vi "Find max pump WP angle.vi"(8 "error in (no error)":errorcluster, 9 "Angle":dbl, 10 "Delay":u32, 11 "VISA Refnum in":refnum<visa-resource-name>) -> (0 "error out":errorcluster, 1 "Numeric":dbl, 2 "Current position (units)":dbl, 3 "VISA Refnum out":refnum<visa-resource-name>)   [LabVIEW 2013]
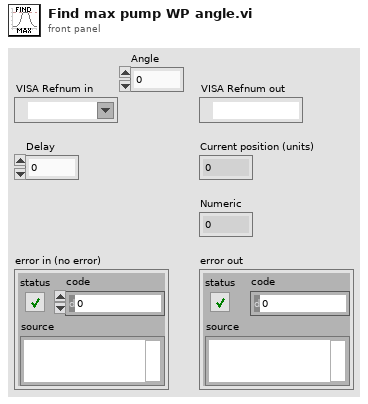
[diagram p1: front panel]
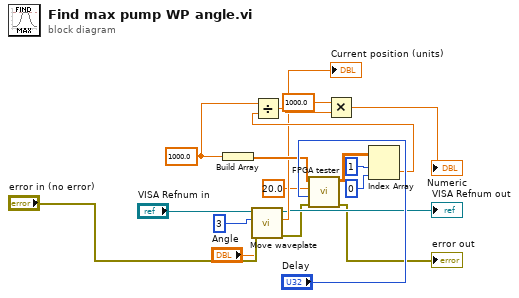
[diagram p0: block diagram]
diagram:
  w14 = 1000.0 ("element")
  n1 = Build Array(w14) -> (w13:dbl[])
  n2 = call "Move waveplate.vi"("error in (no error)"="error in (no error)", "Angle"="Angle", "Axis in"=3, "VISA Refnum in"="VISA Refnum in") -> ("error out"=w8:errorcluster, "Current position (units)"=→"Current position (units)":dbl, "VISA Refnum out"=→"VISA Refnum out":refnum<visa-resource-name>)  [unwired: 4 in, 1 out]
  n3 = call "FPGA tester.vi"("error in"=w8, "Delay"="Delay", "Repetitions"=20.0, "Levels"=w13) -> ("error out"=→"error out":errorcluster, "Results"=w4:dbl[][])  [unwired: 2 in]
  n4 = Index Array(array=w4, index (row)=1, index (col)=0 ("disabled index (col)")) -> (element=w15:dbl)
  n5 = Divide(x=w14, y=w15) -> (x/y=w16:dbl)
  n6 = Multiply(x=1000.0, y=w16) -> (x*y=→"Numeric":dbl)
